vi "Delete directory and send to Recycle Bin.vi"(8 "error in":errorcluster, 9 "Delete Options":i32(ring)=3 items=["DeletePermanently"=2, "SendToRecycleBin"=3], 10 "Dialog Options":i32(ring)=2 items=["OnlyErrorDialogs"=2, "AllDialogs"=3], 11 "Directory to Recycle":path) -> (0 "error out":errorcluster)   [LabVIEW 2013]
uses:
  Microsoft.VisualBasic
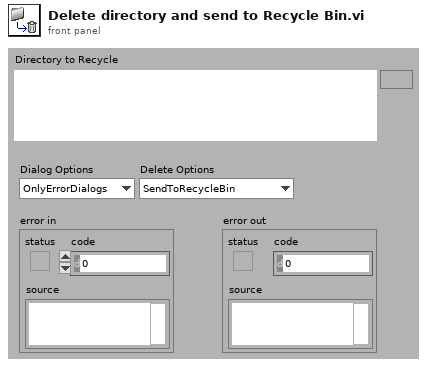
[diagram p1: front panel]
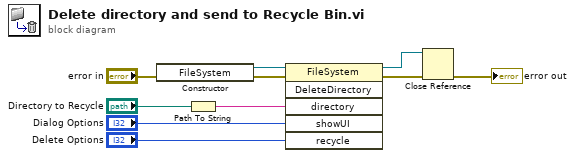
[diagram p0: block diagram]
diagram:
  n1 = constructor class="FileSystem"(error in="error in") -> (reference out=w9:refnum<k24>, error out=w10:errorcluster)  [unwired: 2 in, 1 out]
  n2 = Path To String(path="Directory to Recycle") -> (string=w3:string)
  n3 = invoke class="FileSystem" method="DeleteDirectory"(reference=w9, error in=w10, "directory"=w3, "showUI"="Dialog Options", "recycle"="Delete Options") -> (reference out=w7:refnum<k24>, error out=w6:errorcluster)  [unwired: 1 in, 4 out]
  n4 = Close Reference(reference=w7, error in (no error)=w6) -> (error out=→"error out":errorcluster)
